vi "Destroy Buffer.vi"(8 "error in":errorcluster, 9 "Return Elements (T)":bool=TRUE, 11 "Buffer":refnum<data-value>) -> (0 "error out":errorcluster, 2 "elements":variant[](array[variant]))   [LabVIEW 2013, in "CircularBuffer.lvlib" / "VariantBuffer.lvclass"]
doc: "This VI releases resources that have been created for the ring buffer."
uses:
  VariantBuffer.lvclass
  VariantBuffer.lvclass/VariantBuffer.ctl
  buffer-event -- enum.ctl
  WriteBufferError.vi
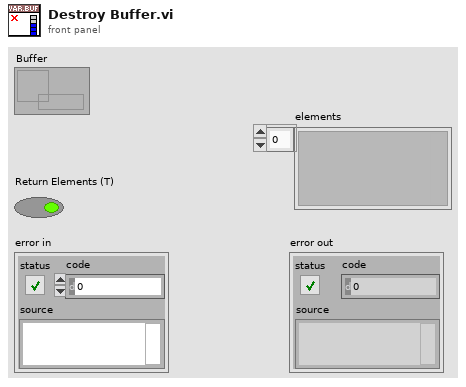
[diagram p1: front panel]
types:
  T1 = typedef "CircularBuffer.lvlib/VariantBuffer.lvclass/buffer-event -- enum.ctl" = enum16{"element-added", "element-removed", "filled", "emptied", "resized", "default-changed", "destroyed"}
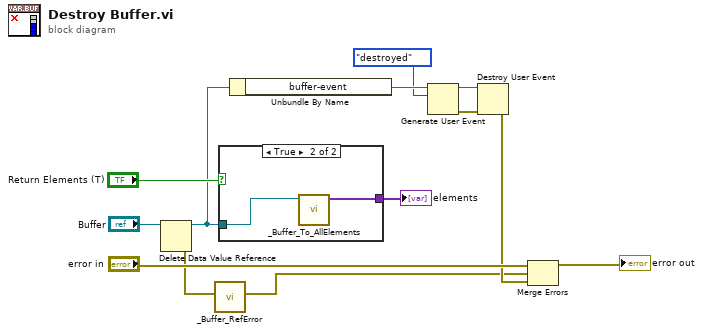
[diagram p0: block diagram]
diagram:
  n1 = Delete Data Value Reference(data value reference="Buffer") -> (data value=w8:refnum<class "VariantBuffer.lvclass">, error out=w2:errorcluster)  [unwired: 1 in]
  n2 = call "_Buffer_RefError.vi"("error in (no error)"=w2) -> ("error out"=w1:errorcluster)  [unwired: 10 in]
  n3 = case shown="True" "Return Elements (T)" {
    tunnel: w8 -> [_ w15]
    tunnel: [_ w14] -> w12
    frame False {
    }
    frame True {
      n4 = call "_Buffer_To_AllElements.vi"("Buffer"=w15) -> ("elements"=w14:variant[])  [unwired: 10 in]
    }
  }
  "elements" <- w12
  n5 = Unbundle By Name(w8) -> ("buffer-event"=w7:refnum<user-event>)
  n6 = Generate User Event(user event=w7, event data cluster=buffer-event_--_enum."destroyed" ("event data")) -> (user event out=w4:refnum<user-event>, error out=w5:errorcluster)  [unwired: 2 in]
  n7 = Destroy User Event(user event=w4, error in=w5) -> (error out=w3:errorcluster)
  n8 = Merge Errors("error in", w1, w3) -> (→"error out":errorcluster)
